vi "read_sample_weight.vi"(8 "error in (no error)":errorcluster, 11 "Naive_bayes in":refnum<class "Naive_bayes.lvclass">) -> (0 "error out":errorcluster, 2 "sample_weight":dbl[](array[numeric]), 3 "Naive_bayes out":refnum<class "Naive_bayes.lvclass">)   [LabVIEW 2020, in "Naive_bayes.lvclass"]
uses:
  Naive_bayes.lvclass
  Naive_bayes.lvclass/Naive_bayes.ctl
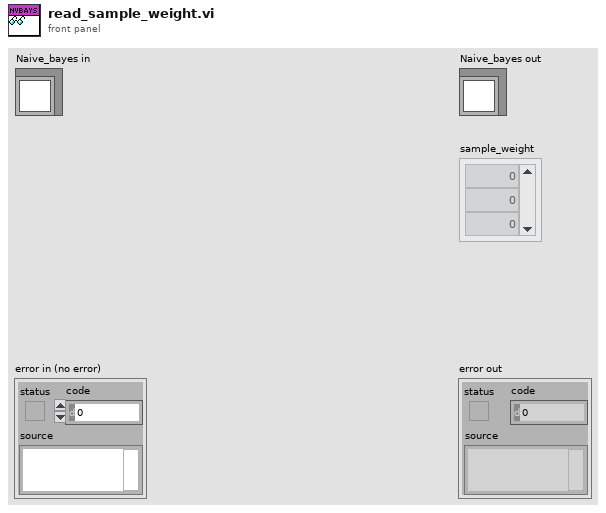
[diagram p1: front panel]
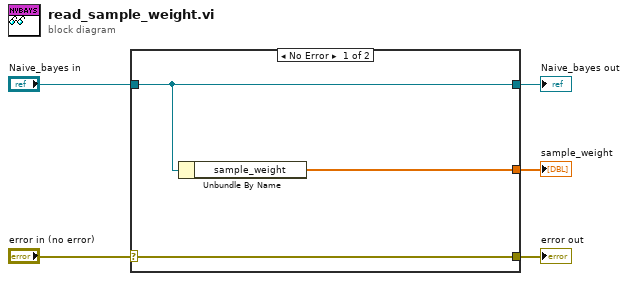
[diagram p0: block diagram]
diagram:
  n1 = case shown="No Error" "error in (no error)" {
    selector: "error in (no error)" -> [w8 w9]
    tunnel: [w8 w9] -> w4
    tunnel: [w7 w10] -> w2
    tunnel: "Naive_bayes in" -> [w7 w10]
    tunnel: [w6 _] -> w1
    frame No Error {
      n2 = Unbundle By Name(w7) -> ("sample_weight"=w6:dbl[])
    }
    frame Error {
    }
  }
  "error out" <- w4
  "Naive_bayes out" <- w2
  "sample_weight" <- w1
